vi "pump_control.vi"(0 "VISA resource name":refnum<visa-resource-name>="ASRL1::INSTR", 1 "Direction":u16(ring) items=["Infuse", "Withdraw", "No Action"], 2 "Syringe Inside Diameter (19.58 mm)\nIf diameter is upper than 14.00 mm : Volume units are mL\nIf diameter is lower than 14.00 mm : Volume units are µL":dbl=19.58 min=0.1 max=50.0 step=0.01 format="%#_4g", 3 "Dispense Volume (mL)":dbl=1.5 format="%_6f", 4 "Units":i32(ring)=2 items=["microliters per minute (µL/min)", "microliters per hour (µL/hr)", "milliliters per minute (mL/min)", "milliliters per hour (mL/hr)"], 5 "Flow rate":dbl=5.0 format="%.3f") -> (6 "Pump : New Era Pump Systems Inc.\nFirmware Version :":string, 7 "Volume Dispensed":string, 8 "Pump Status":T1)   [LabVIEW 2019]
uses:
  <vilib>/Utility/error.llb/DialogType.ctl
panel:
  in  "Pump Address (0)":i32 format="%0#.0f"
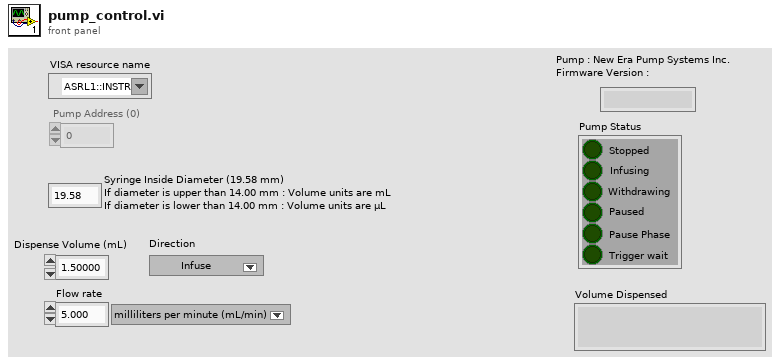
[diagram p1: front panel]
types:
  T1 = cluster{"Stopped":bool, "Infusing":bool, "Withdrawing":bool, "Paused":bool, "Pause Phase":bool, "Trigger wait":bool}
  T2 = typedef "DialogType.ctl" = u16
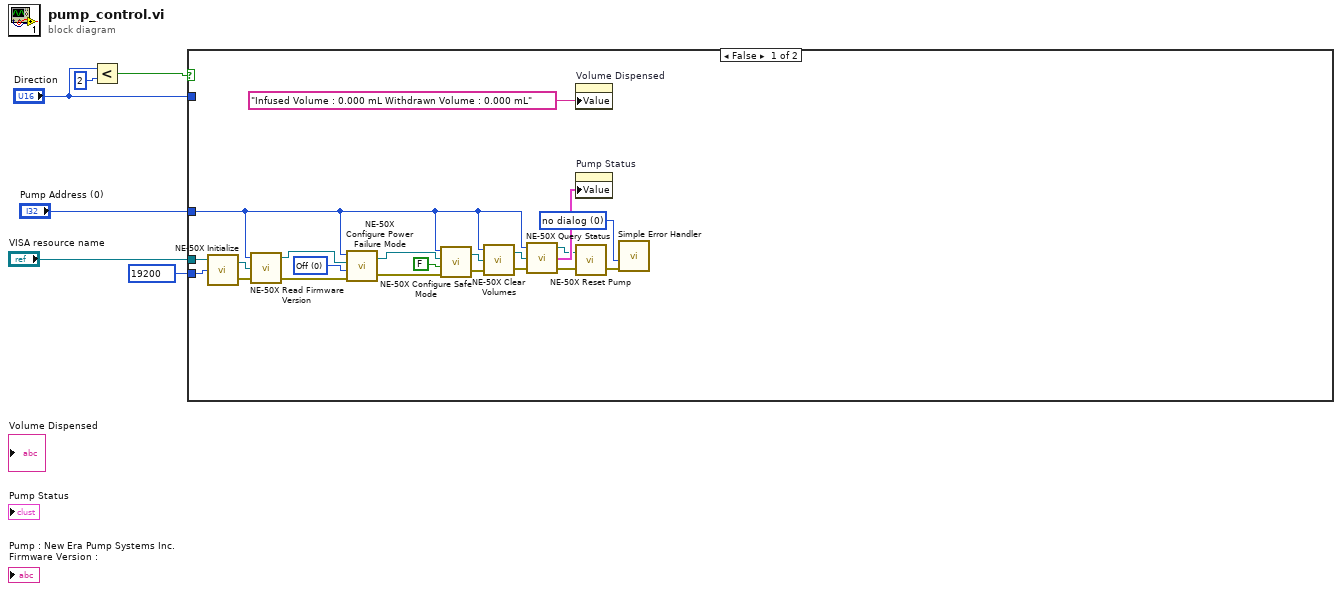
[diagram p0: block diagram]
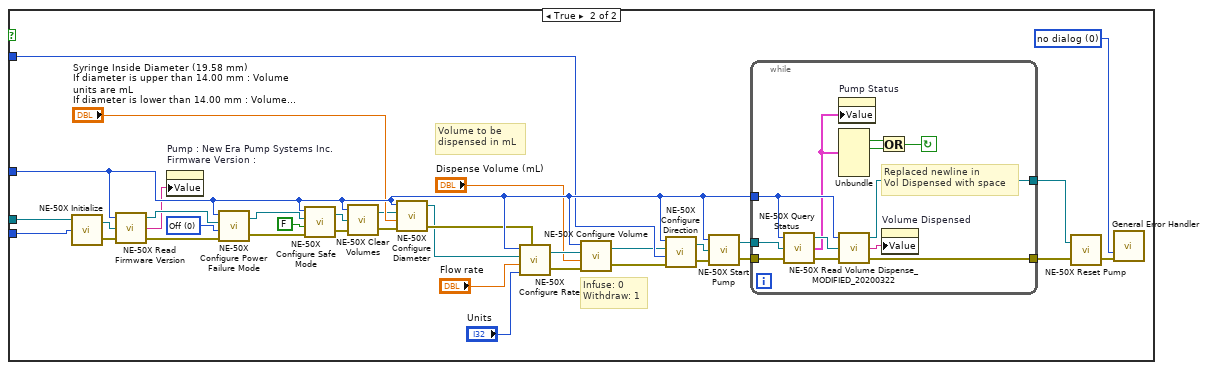
[diagram p2: hidden frame]
diagram:
  w5 = u32 19200 items=["19200"=19200, "9600"=9600, "2400"=2400, "1200"=1200, "300"=300] ("Baud Rate (19200)")
  n1 = Less?(x="Direction", y=2) -> (x < y?=w1:bool)
  n2 = case shown="False" w1 {
    tunnel: "VISA resource name" -> [w13 w62]
    tunnel: w5 -> [w12 w61]
    tunnel: "Pump Address (0)" -> [w7 w60]
    tunnel: "Direction" -> [_ w59]
    frame False {
      w14 = T2 0 items=["no dialog", "OK message", "continue or stop message", "OK message + warnings", "continue/stop + warnings"] ("type of dialog (OK msg:1)")
      w20 = u16 0 items=["Off", "On"] ("0 = Disabled")
      n3 = call "NE-50X Initialize.vi"("Baud Rate (19200)"=w12, "VISA resource name"=w13) -> ("error out"=w27:errorcluster, "VISA resource name out"=w18:refnum<visa-resource-name>)  [unwired: 1 in]
      n4 = call "NE-50X Read Firmware Version.vi"("error in (no error)"=w27, "VISA resource name"=w18, "Address (0)"=w7) -> ("error out"=w26:errorcluster, "VISA resource name out"=w19:refnum<visa-resource-name>)  [unwired: 1 out]
      n5 = call "NE-50X Configure Power Failure Mode.vi"("error in (no error)"=w26, "Power Failure Mode"=w20, "VISA resource name"=w19, "Address (0)"=w7) -> ("error out"=w25:errorcluster, "VISA resource name out"=w21:refnum<visa-resource-name>)
      n6 = call "NE-50X Configure Safe Mode.vi"("error in (no error)"=w25, "Safe Mode"=FALSE ("0 = Basic"), "VISA resource name"=w21, "Address (0)"=w7) -> ("error out"=w23:errorcluster, "VISA resource name out"=w22:refnum<visa-resource-name>)
      n7 = call "NE-50X Clear Volumes.vi"("error in (no error)"=w23, "VISA resource name"=w22, "Address (0)"=w7) -> ("error out"=w16:errorcluster, "VISA resource name out"=w17:refnum<visa-resource-name>)
      n8 = call "NE-50X Query Status.vi"("error in (no error)"=w16, "VISA resource name"=w17, "Address (0)"=w7) -> ("error out"=w10:errorcluster, "Status"=w11:T1, "VISA resource name out"=w9:refnum<visa-resource-name>)
      n9 = property on="Volume Dispensed" class="Str"("Value"="Infused Volume : 0.000 mL Withdrawn Volume : 0.000 mL" ("Volume Dispensed")) -> ()  [unwired: 2 in, 2 out]
      n10 = property on="Pump Status" class="Clust (strict)"("Value"=w11) -> ()  [unwired: 2 in, 2 out]
      n11 = call "NE-50X Reset Pump.vi"("error in (no error)"=w10, "VISA resource name"=w9) -> ("error out"=w15:errorcluster)  [unwired: 1 out]
      n12 = call <vilib>:"Simple Error Handler.vi"("type of dialog (OK msg:1)"=w14, "error in (no error)"=w15) -> ()  [unwired: 3 in, 5 out]
    }
    frame True {
      w32 = T2 0 items=["no dialog", "OK message", "continue or stop message", "OK message + warnings", "continue/stop + warnings"] ("type of dialog (OK msg:1)")
      w40 = u16 0 items=["Off", "On"] ("0 = Disabled")
      # "Infuse: 0\nWithdraw: 1"
      # "Volume to be \ndispensed in mL"
      n13 = call "NE-50X Initialize.vi"("Baud Rate (19200)"=w61, "VISA resource name"=w62) -> ("error out"=w57:errorcluster, "VISA resource name out"=w38:refnum<visa-resource-name>)  [unwired: 1 in]
      n14 = call "NE-50X Read Firmware Version.vi"("error in (no error)"=w57, "VISA resource name"=w38, "Address (0)"=w60) -> ("error out"=w56:errorcluster, "Version"=w28:string, "VISA resource name out"=w39:refnum<visa-resource-name>)
      n15 = property on="Pump : New Era Pump Systems Inc.\nFirmware Version :" class="Str"("Value"=w28) -> ()  [unwired: 2 in, 2 out]
      n16 = call "NE-50X Configure Power Failure Mode.vi"("error in (no error)"=w56, "Power Failure Mode"=w40, "VISA resource name"=w39, "Address (0)"=w60) -> ("error out"=w55:errorcluster, "VISA resource name out"=w41:refnum<visa-resource-name>)
      n17 = call "NE-50X Configure Safe Mode.vi"("error in (no error)"=w55, "Safe Mode"=FALSE ("0 = Basic"), "VISA resource name"=w41, "Address (0)"=w60) -> ("error out"=w51:errorcluster, "VISA resource name out"=w42:refnum<visa-resource-name>)
      n18 = call "NE-50X Clear Volumes.vi"("error in (no error)"=w51, "VISA resource name"=w42, "Address (0)"=w60) -> ("error out"=w58:errorcluster, "VISA resource name out"=w43:refnum<visa-resource-name>)
      n19 = call "NE-50X Configure Diameter.vi"("error in (no error)"=w58, "Diameter (19.58 mm)"="Syringe Inside Diameter (19.58 mm)\nIf diameter is upper than 14.00 mm : Volume units are mL\nIf diameter is lower than 14.00 mm : Volume units are µL", "VISA resource name"=w43, "Address (0)"=w60) -> ("error out"=w50:errorcluster, "VISA resource name out"=w44:refnum<visa-resource-name>)  [unwired: 1 out]
      n20 = call "NE-50X Configure Rate.vi"("Address (0)"=w60, "VISA resource name"=w44, "Flow"="Flow rate", "Units"="Units", "error in (no error)"=w50) -> ("VISA resource name out"=w45:refnum<visa-resource-name>, "error out"=w52:errorcluster)
      n21 = call "NE-50X Configure Volume.vi"("error in (no error)"=w52, "Volume"="Dispense Volume (mL)", "VISA resource name"=w45, "Address (0)"=w60) -> ("error out"=w53:errorcluster, "VISA resource name out"=w46:refnum<visa-resource-name>)
      n22 = call "NE-50X Configure Direction.vi"("error in (no error)"=w53, "Direction"=w59, "VISA resource name"=w46, "Address (0)"=w60) -> ("error out"=w37:errorcluster, "VISA resource name out"=w36:refnum<visa-resource-name>)
      n23 = call "NE-50X Start Pump.vi"("error in (no error)"=w37, "VISA resource name"=w36, "Address (0)"=w60) -> ("error out"=w34:errorcluster, "VISA resource name out"=w33:refnum<visa-resource-name>)
      n24 = while {
        tunnel: w60 -> [w67]
        tunnel: w33 -> [w73]
        tunnel: [w66] -> w30
        tunnel: w34 -> [w74]
        tunnel: [w68] -> w29
        stop <- w65 continue-if-true
        # "Replaced newline in\nVol Dispensed with space"
        n25 = call "NE-50X Query Status.vi"("error in (no error)"=w74, "VISA resource name"=w73, "Address (0)"=w67) -> ("error out"=w72:errorcluster, "Status"=w64:T1, "VISA resource name out"=w71:refnum<visa-resource-name>)
        n26 = property on="Pump Status" class="Clust (strict)"("Value"=w64) -> ()  [unwired: 2 in, 2 out]
        n27 = Unbundle(w64) -> ("Infusing"=w70:bool, "Withdrawing"=w69:bool)  [unwired: 4 out]
        n28 = call "NE-50X Read Volume Dispense_MODIFIED_20200322.vi"("error in (no error)"=w72, "VISA resource name"=w71, "Address (0)"=w67) -> ("error out"=w68:errorcluster, "Volume Dispense"=w63:string, "VISA resource name out"=w66:refnum<visa-resource-name>)
        n29 = Or(x=w70, y=w69) -> (x .or. y?=w65:bool)
        n30 = property on="Volume Dispensed" class="Str"("Value"=w63) -> ()  [unwired: 2 in, 2 out]
      }
      n31 = call "NE-50X Reset Pump.vi"("error in (no error)"=w29, "VISA resource name"=w30) -> ("error out"=w31:errorcluster)  [unwired: 1 out]
      n32 = call <vilib>:"General Error Handler.vi"("type of dialog (OK msg:1)"=w32, "error in (no error)"=w31) -> ()  [unwired: 9 in, 5 out]
    }
  }
